vi "Collect Lift Gain Scheduler.vi"(11 "Collector Lift States":T1) -> (3 "Collect Lift Gains Out":cluster{"kP":dbl, "kI":dbl, "kD":dbl})   [LabVIEW 2015]
uses:
  Typedefs/CollectorLiftStates.ctl
panel:
  in  "Collector Lift Gains":cluster{"kP":dbl, "kI":dbl, "kD":dbl}[](array[cluster])=[{"kP"=0.0, "kI"=0.0, "kD"=0.0}, {"kP"=0.0, "kI"=0.0, "kD"=0.0}, {"kP"=0.0, "kI"=0.0, "kD"=0.0}, {"kP"=0.0, "kI"=0.0, "kD"=0.0}]
  # "Normal"
  # "CDF"
  # "Manual"
  # "Portcullis"
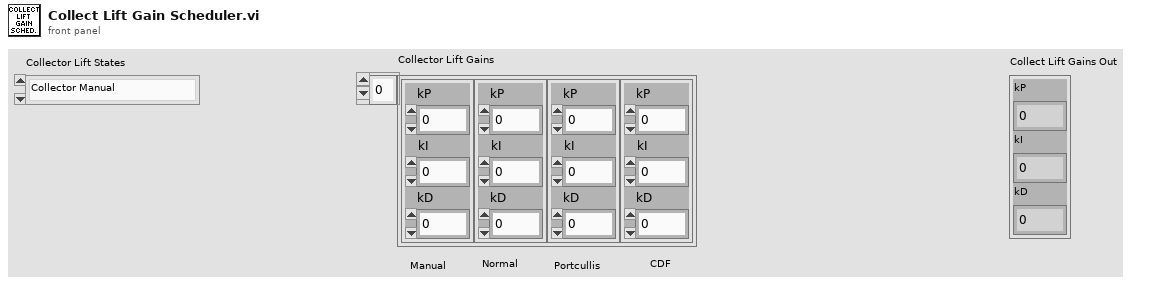
[diagram p1: front panel]
types:
  T1 = typedef "CollectorLiftStates.ctl" = enum16{"Collector Manual", "Stow", "Collect Position", "Spit Position", "Portcullis Set Up", "Portcullis Lift Up", "CDF Set Up", "Push CDF Down"}
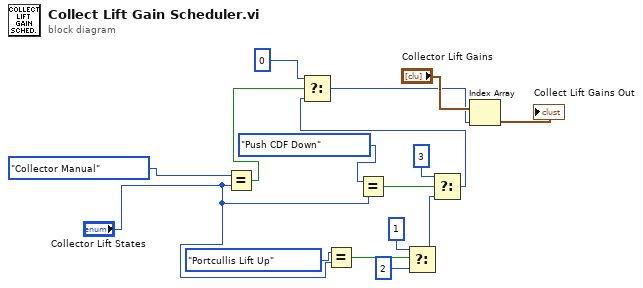
[diagram p0: block diagram]
diagram:
  n1 = Equal?(x=CollectorLiftStates."Collector Manual" ("Collector Lift States 2"), y="Collector Lift States") -> (x = y?=w11:bool)
  n2 = Equal?(x=CollectorLiftStates."Portcullis Lift Up" ("Collector Lift States 2"), y="Collector Lift States") -> (x = y?=w4:bool)
  n3 = Equal?(x=CollectorLiftStates."Push CDF Down" ("Collector Lift States 2"), y="Collector Lift States") -> (x = y?=w8:bool)
  n4 = Select(t=i8 1, s=w4, f=i8 2) -> (s? t:f=w5:i8)
  n5 = Select(t=i8 3, s=w8, f=w5) -> (s? t:f=w6:i8)
  n6 = Select(t=i8 0, s=w11, f=w6) -> (s? t:f=w2:i8)
  n7 = Index Array(array="Collector Lift Gains", index=w2) -> (element=→"Collect Lift Gains Out":cluster{"kP":dbl, "kI":dbl, "kD":dbl})
